vi "PAQmem_FindStartTimeIndex.vi"(8 "error in (no error)":errorcluster, 10 "Start-time":timestamp, 11 "PAQ-memory in":refnum<class "PAQ-memory.lvclass">) -> (0 "error out":errorcluster, 1 "Size":i32, 2 "Start":i32, 3 "PAQ-memory out":refnum<class "PAQ-memory.lvclass">, 4 "time":timestamp[](array[timestamp]))   [LabVIEW 2020, in "Sgraph_lib_V1.lvlib" / "PAQ-memory.lvclass"]
doc: "Andre Koelewijn, 17 Jan 2021\n\nFind the index of the start time when searching for the last PAQ buffer section"
uses:
  PAQ-memory.lvclass
  PAQ-memory.lvclass/PAQ-memory.ctl
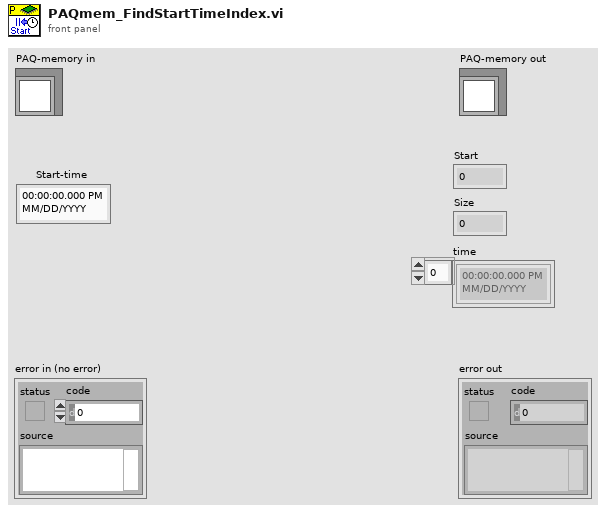
[diagram p1: front panel]
types:
  T1 = typedef "Sgraph_lib_V1.lvlib/FAMM.lvclass/typedef_PAQdata.ctl" = cluster{"TAGs":string[], "Time":refnum<data-value>, "TAGdata":cluster{"source":refnum<data-value>, "status":refnum<data-value>, "data":refnum<data-value>, "max":refnum<data-value>, "min":refnum<data-value>}[]}
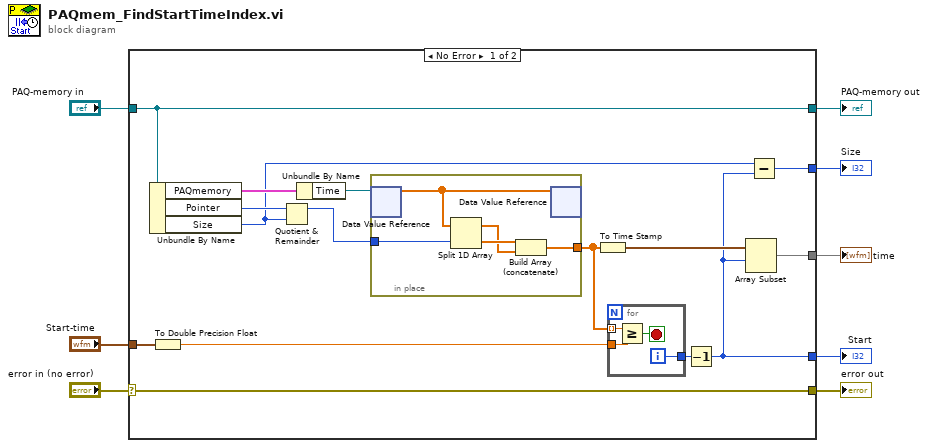
[diagram p0: block diagram]
diagram:
  n1 = case shown="No Error" "error in (no error)" {
    selector: "error in (no error)" -> [w23 w34]
    tunnel: [w23 w34] -> w7
    tunnel: [w20 w33] -> w5
    tunnel: "PAQ-memory in" -> [w20 w33]
    tunnel: [w13 _] -> w1
    tunnel: "Start-time" -> [w17 _]
    tunnel: [w9 _] -> w3
    tunnel: [w10 _] -> w2
    frame No Error {
      n2 = Unbundle By Name(w20) -> ("PAQmemory"=w22:T1, "Pointer"=w18:i32, "Size"=w12:i32)
      n3 = To Double Precision Float(number=w17) -> (double precision float=w15:dbl)
      n4 = Quotient & Remainder(x=w18, y=w12) -> (x-y*floor(x/y)=w19:i32)  [unwired: 1 out]
      n5 = Unbundle By Name(w22) -> ("Time"=w21:refnum<data-value>)
      n6 = in-place {
        in-place-border: w19 -> [w31]
        in-place-border: [w28] -> w16
        n7 = in-place-dvr #1(w21) -> (w32:dbl[])  [unwired: 1 out]
        n8 = Split 1D Array(array=w32, index=w31) -> (first subarray=w29:dbl[], second subarray=w30:dbl[])
        n9 = Build Array (concatenate)(w30, w29) -> (w28:dbl[])
        n10 = in-place-dvr #1(w32) -> ()  [unwired: 2 out]
      }
      n11 = To Time Stamp(1:w16) -> (0:w14:timestamp[])
      n12 = for {
        tunnel: w16 -> [w27] mode=indexing
        tunnel: w15 -> [w26]
        tunnel: [w24] -> w11
        i -> [w24]
        stop <- w25 stop-if-true
        n13 = Greater Or Equal?(x=w27, y=w26) -> (x >= y?=w25:bool)
      }
      n14 = Decrement(x=w11) -> (x-1=w9:i32)
      n15 = Array Subset(array=w14, index=w9) -> (w13:timestamp[])  [unwired: 1 in]
      n16 = Subtract(x=w12, y=w9) -> (x-y=w10:i32)
    }
    frame Error {
    }
  }
  "error out" <- w7
  "PAQ-memory out" <- w5
  "time" <- w1
  "Start" <- w3
  "Size" <- w2
